vi "SSC DCPower Get Source Adapt Settings.vi"(0 "DCPower SSC in":T2[](array[typedef]), 11 "error in":errorcluster) -> (4 "DCPower SSC out":T2[](array[typedef]), 6 "Voltage":T1[](array[typedef]) {"Pole-Zero Ratio" format="%#_6p"; "Compensation Frequency" format="%#_6p"; "Gain Bandwidth" format="%#_6p"}, 8 "Current":T1[](array[typedef]) {"Pole-Zero Ratio" format="%#_6p"; "Compensation Frequency" format="%#_6p"; "Gain Bandwidth" format="%#_6p"}, 10 "Transient Response":i32[](array[ring]) items=["Slow"=1041, "Normal"=1038, "Fast"=1039, "Custom"=1042], 15 "error out":errorcluster)   [LabVIEW 2020]
doc: "This VI gets the transient response settings (e.g. Source Adapt parameters) for the channels.\n\nThis can be used to get the source adapt parameters for the default transient response settings (Slow, Normal, Fast) if the channels are in those modes."
uses:
  SSC DCPower.ctl
  SSC DCPower Source Adapt.ctl
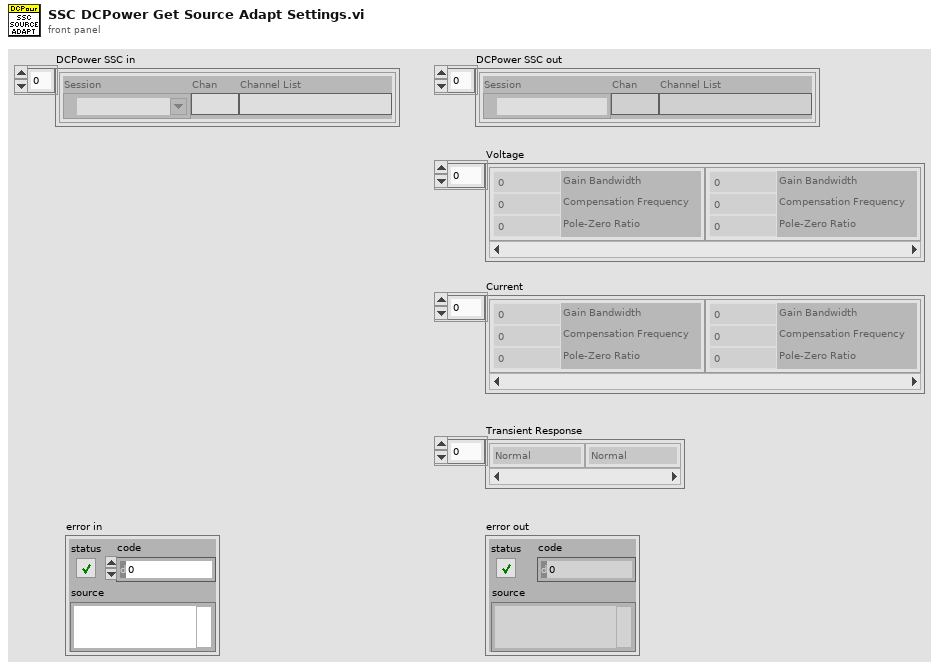
[diagram p1: front panel]
types:
  T1 = typedef "SSC DCPower Source Adapt.ctl" = cluster{"Gain Bandwidth":dbl, "Compensation Frequency":dbl, "Pole-Zero Ratio":dbl}
  T2 = typedef "SSC DCPower.ctl" = cluster{"Session":refnum<k15>, "Chan":string, "Channel List":string}
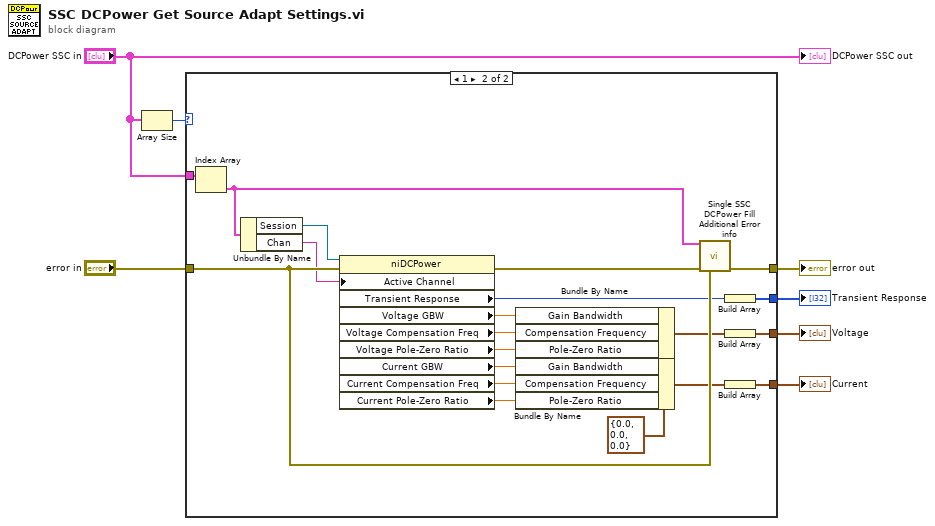
[diagram p0: block diagram]
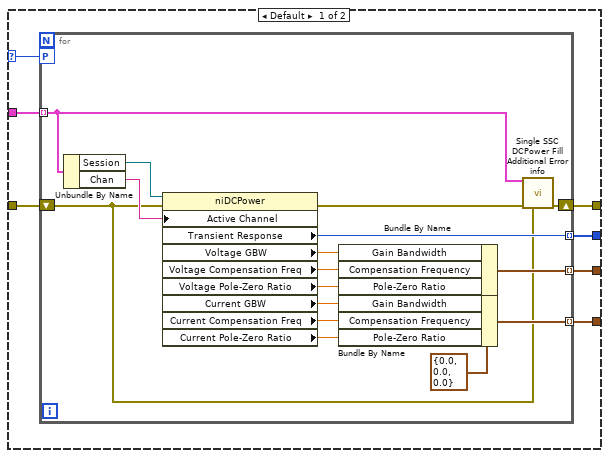
[diagram p2: hidden frame]
diagram:
  n1 = Array Size(array="DCPower SSC in") -> (size(s)=w2:i32)
  n2 = case shown="1" w2 {
    selector: w2 -> [w9 _]
    tunnel: [w14 w50] -> w7
    tunnel: "error in" -> [w13 w49]
    tunnel: [w12 w32] -> w5
    tunnel: [w11 w31] -> w4
    tunnel: [w10 w33] -> w3
    tunnel: "DCPower SSC in" -> [w8 w45]
    frame Default {
      n3 = for {
        tunnel: w8 -> [w16] mode=indexing
        workers-P: w9 -> [_]
        tunnel: [w29] -> w12 mode=indexing
        tunnel: [w28] -> w11 mode=indexing
        tunnel: [w27] -> w10 mode=indexing
        shift-right: [w17] -> w14
        shift-left: w13 -> [w15]
        w18 = T1 {"Gain Bandwidth"=0.0, "Compensation Frequency"=0.0, "Pole-Zero Ratio"=0.0} ("Current")
        n4 = Unbundle By Name(w16) -> ("Session"=w26:refnum<k15>, "Chan"=w25:string)
        n5 = property class="niDCPower"(reference=w26, error in=w15, "Active Channel"=w25) -> (error out=w30:errorcluster, "Transient Response"=w27:i32, "Voltage GBW"=w24:dbl, "Voltage Compensation Freq"=w23:dbl, "Voltage Pole-Zero Ratio"=w22:dbl, "Current GBW"=w21:dbl, "Current Compensation Freq"=w20:dbl, "Current Pole-Zero Ratio"=w19:dbl)  [unwired: 1 out]
        n6 = Bundle By Name(cluster=w18, "Gain Bandwidth"=w24, "Compensation Frequency"=w23, "Pole-Zero Ratio"=w22) -> (w29:T1)
        n7 = Bundle By Name(cluster=w18, "Gain Bandwidth"=w21, "Compensation Frequency"=w20, "Pole-Zero Ratio"=w19) -> (w28:T1)
        n8 = call "Single SSC DCPower Fill Additional Error info.vi"("DCPower SSC in"=w16, "error in"=w30, "previous error in"=w15) -> ("error out"=w17:errorcluster)  [unwired: 12 in]
      }
    }
    frame 1 {
      w35 = T1 {"Gain Bandwidth"=0.0, "Compensation Frequency"=0.0, "Pole-Zero Ratio"=0.0} ("Current")
      n9 = Index Array(array=w45) -> (element=w34:T2)  [unwired: 1 in]
      n10 = Unbundle By Name(w34) -> ("Session"=w43:refnum<k15>, "Chan"=w42:string)
      n11 = property class="niDCPower"(reference=w43, error in=w49, "Active Channel"=w42) -> (error out=w44:errorcluster, "Transient Response"=w46:i32, "Voltage GBW"=w41:dbl, "Voltage Compensation Freq"=w40:dbl, "Voltage Pole-Zero Ratio"=w39:dbl, "Current GBW"=w38:dbl, "Current Compensation Freq"=w37:dbl, "Current Pole-Zero Ratio"=w36:dbl)  [unwired: 1 out]
      n12 = Bundle By Name(cluster=w35, "Gain Bandwidth"=w41, "Compensation Frequency"=w40, "Pole-Zero Ratio"=w39) -> (w48:T1)
      n13 = Bundle By Name(cluster=w35, "Gain Bandwidth"=w38, "Compensation Frequency"=w37, "Pole-Zero Ratio"=w36) -> (w47:T1)
      n14 = call "Single SSC DCPower Fill Additional Error info.vi"("DCPower SSC in"=w34, "error in"=w44, "previous error in"=w49) -> ("error out"=w50:errorcluster)  [unwired: 12 in]
      n15 = Build Array(w46) -> (w33:i32[])
      n16 = Build Array(w48) -> (w32:T1[])
      n17 = Build Array(w47) -> (w31:T1[])
    }
  }
  "error out" <- w7
  "Current" <- w4
  "Voltage" <- w5
  "Transient Response" <- w3
  "DCPower SSC out" <- "DCPower SSC in"
